vi "VSS Vision Log Player.vi"() -> ()   [LabVIEW 2018]
uses:
  GUI/IA Robot Line Display.ctl
  Intel/Functions Enum.ctl
  Filters/Estimadores.ctl
  Control/SSL Data Control.ctl
  Control/SSL UDP Address.ctl
  Control/File Player.ctl
  Intel/Command Enum.ctl
  Test/TestModule.ctl
  Util/Select None or Robot.ctl
  DrawTargets.ctl
  Select Personalitys.ctl
  Util/Select Auto None or Robot.ctl
  Intel/AI Parameters.ctl
  SSL Referee Game Status.ctl
  SSL/VSS Field State.ctl
  SSL Detection Frame.ctl
  SSL Detection Robot.ctl
  <vilib>/Analysis/Matrix/Datatypes/RealMatrix.ctl
  SSL Detection Ball.ctl
  <extravilib>/ChannelInstances/Lossy Stream-t'AI Input.ctl'/Read With Abort.vi
  <extravilib>/ChannelInstances/Lossy Stream-bool/Write With Abort.vi
  <extravilib>/ChannelInstances/Lossy Stream-a[.](u8)/Read With Abort.vi
  <extravilib>/ChannelInstances/Lossy Stream-t'VSS Field State.ctl'/Write With Abort.vi
  <extravilib>/ChannelInstances/Lossy Stream-bool/Read With Abort.vi
  <extravilib>/ChannelInstances/Lossy Stream-t'VSS Field State.ctl'/Read With Abort.vi
  <extravilib>/ChannelInstances/Lossy Stream-a[.](u16)/Write With Abort.vi
  <extravilib>/ChannelInstances/Lossy Stream-t'AI Input.ctl'/Write With Abort.vi
  <extravilib>/ChannelInstances/Lossy Stream-t'AI Input.ctl'/EndpointRead.vi
  <extravilib>/ChannelInstances/Lossy Stream-bool/Endpoint.vi
  <extravilib>/ChannelInstances/Lossy Stream-a[.](u8)/EndpointRead.vi
  <extravilib>/ChannelInstances/Lossy Stream-t'VSS Field State.ctl'/Endpoint.vi
  <extravilib>/ChannelInstances/Lossy Stream-bool/EndpointRead.vi
  <extravilib>/ChannelInstances/Lossy Stream-t'VSS Field State.ctl'/EndpointRead.vi
  <extravilib>/ChannelInstances/Lossy Stream-a[.](u16)/Endpoint.vi
  <extravilib>/ChannelInstances/Lossy Stream-t'AI Input.ctl'/Endpoint.vi
  <extravilib>/ChannelInstances/Lossy Stream-bool/Instantiate.vi
  <extravilib>/ChannelInstances/Lossy Stream-a[.](u8)/Instantiate.vi
  <extravilib>/ChannelInstances/Lossy Stream-t'VSS Field State.ctl'/Instantiate.vi
  <extravilib>/ChannelInstances/Lossy Stream-a[.](u16)/Instantiate.vi
  <extravilib>/ChannelInstances/Lossy Stream-t'AI Input.ctl'/Instantiate.vi
  <extravilib>/ChannelInstances/Lossy Stream-bool/)Channel.vi
  <resource>/ChannelSupport/_ChannelSupport/WaitIfNeeded.vi
  <extravilib>/ChannelInstances/Lossy Stream-t'VSS Field State.ctl'/)Channel.vi
  <extravilib>/ChannelInstances/Lossy Stream-a[.](u16)/)Channel.vi
  <extravilib>/ChannelInstances/Lossy Stream-t'AI Input.ctl'/)Channel.vi
  <extravilib>/ChannelInstances/Lossy Stream-a[.](u8)/)Channel.vi
  Util/PreviousState.vi
  <extravilib>/ChannelInstances/Lossy Stream-t'AI Input.ctl'.lvlib
  <extravilib>/ChannelInstances/Lossy Stream-a[.](u8).lvlib
  <vilib>/Analysis/Matrix/NI_Matrix.lvlib
  <extravilib>/ChannelInstances/Lossy Stream-t'VSS Field State.ctl'.lvlib
  <extravilib>/ChannelInstances/Lossy Stream-a[.](u16).lvlib
  <extravilib>/ChannelInstances/Lossy Stream-bool.lvlib
panel:
  in  "Personalidade Dinâmica":bool
  in  "element":T1={"Stage"="First Half", "Command"="Stop", "Time Left"=0.0, "Yellow Team"="", "Blue Team"="", "Yellow Score"=0, "Blue Score"=0, "Yellow Red Cards"=0, "Blue Red Cards"=0, "Yellow Yellow Cards"=0, "Blue Yellow Cards"=0, "Yellow Timeouts Left"=0, "Blue Timeouts Left"=0, "Yellow Timeout Remaining"=0.0, "Blue Timeout Remaining"=0.0, "Yellow Goalie Id"=0, "Blue Goalie Id"=0, "Time"=timestamp(0 s since 1904-01-01)} {"Time" format="%<%.3X %x>T"; "Blue Timeout Remaining" format="%<%M:%S>t"; "Yellow Timeout Remaining" format="%<%M:%S>t"; "Time Left" format="%<%M:%S>t"}
  in  "SSL Vision":bool
  out "Role Playing \nFPS 2":dbl
  in  "Debug":bool
  in  "GoTo Navigation":bool
  out "kick error":dbl
  in  "Pinned":T2={"Attc"="1", "Goal"="4", "Def"="2"}
  in  "Draw Targets?":T4={"Attacker"=TRUE, "Striker"=TRUE, "Goalie"=TRUE, "Defender"=TRUE, "kick"=TRUE, "Est Ball"=TRUE, "Est Robot"=FALSE, "Path S"=FALSE, "Path C"=FALSE}
  in  "SSL Data":T5={"Modo"=TRUE, "VSS Friend & ball UDP RX"={"Port:"=10006, "Server IP:"="224.5.23.2", "Local IP:"="192.168.0.101", "RX"=TRUE}, "VSS Enemy UDP RX"={"Port:"=10006, "Server IP:"="224.5.23.2", "Local IP:"="192.168.0.101", "RX"=TRUE}, "Reprodução de Arquivo"={"file path (use dialog)"=path "E:/Media/2016-07-01_cmdragons_immortals.log", "size (in bytes)"=0, "offset (in bytes)"=0, "Slide"=0.0, "Play"=FALSE, "Time Stamp"=timestamp(0 s since 1904-01-01), "Playing"=FALSE}} {"Reprodução de Arquivo"."Time Stamp" format="%<%.3X %x>T"; "Reprodução de Arquivo"."Slide" min=0 max=1 scale=0.0..1.0; "Reprodução de Arquivo"."offset (in bytes)" format="%.3p"; "Reprodução de Arquivo"."size (in bytes)" format="%.3p"}
  out "error out 5":errorcluster
  in  "IA command":T8
  in  "ignora esquerda?":bool
  in  "ignora lado?":bool
  in  "atacando ao contrário?":bool
  in  "Estimador":T9=enum."Kalman"
  out "Role Playing \nFPS":dbl
  out "Total Delay":dbl format="%#.5g"
  in  "Time":enum16{"Azul", "Amarelo"}(ring)=enum."Amarelo" caption="Enum"
  in  "Lado":enum16{"Esquerdo", "Direito"}(ring)=enum."Direito" caption="Enum"
  in  "Role Decisor":enum16{"Simple Role Decisor", "No Role Decisor"}(ring)
  out "wheel 2":dbl(graph)
  out "wheel 1":dbl(graph)
  in  "Test Module":T10={"Goto"="None", "ZigZag 0"="None", "Kicker"="None", "Vel_kick"=100.0, "Kick"=FALSE, "Modo Teste?"=FALSE, "GoTo point"=[], "zigzag points"=[{"x"=666.0, "y"=0.0}, {"x"=-666.0, "y"=0.0}], "robot id vel"=5, "Dribble"=FALSE, "Gravando"=FALSE, "output xy"=2.0, "output angle"=4.0, "angle zigzag"=0.0}
  in  "Tab Control":enum32{"RX Info", "TX info", "AI Parameters"}(tab)
  out "GUI Robot Array":T12[](array[typedef])
  in  "Serial TX":bool
  in  "UDP GrSim TX":bool=TRUE
  in  "Address:":string="192.168.0.106"
  in  "Port:":u16=10020
  in  "Porta:":refnum<visa-resource-name>
  out "Comm FPS":dbl
  in  "AI Parameters":T14={"GotoKick"={"Dist do cone a frente"=0.0, "attacker farback"=1000.0, "Perto"=300.0, "min dist to kick"=120.0, "kick eps"=0.1, "Time to transition"=0.3}, "Attacker"={"CC chute"=0.55, "CC passe"=0.4, "Kick Force"=100.0, "D ball-robot Kick"=300.0, "D ball-robot Pass"=350.0}, "Defender"={"D max"=1700.0, "Vel p/ robô av"=3.0, "Kick Force"=100.0, "D atk-def"=400.0, "D farback"=300.0}, "Timeout"={"Field/v in x"=6.0, "Dist Robots"=300, "Dist up in y"=300}, "Pose Striker"={"dist"=650.0, "Numeric"=-4.0, "dist 2"=650.0}, "Dist Stop"=300.0, "Distance when ball out"=200, "D central gap "=125.0, "T pass"=5.0, "Force ++"=100.0, "range kick"=50.0, "Chute alto"=TRUE, "Marcador novo"=TRUE} {"D central gap" format="%#_13g"; "Dist Stop" format="%#_13g"; "Pose Striker"."Numeric" format="%#_13g"; "Defender"."Kick Force" format="%#_13g"; "Defender"."Vel p/ robô av" format="%#_13g"; "Attacker"."D ball-robot Kick" format="%#_13g"; "Attacker"."Kick Force" format="%#_13g"; "Attacker"."CC passe" format="%#_13g"; "Attacker"."CC chute" format="%#_13g"; "GotoKick"."min dist to kick" format="%#_13g"; "GotoKick"."Perto" format="%#_13g"; "GotoKick"."attacker farback" format="%#_13g"; "GotoKick"."Dist do cone a frente" format="%#_13g"}
  in  "Dist posse":dbl=220.0
  in  "Tol ang posse":dbl=0.3
  in  "Dist Toque":dbl=130.0
  in  "Qtd Min p/ Stk":dbl=2.0
  # "Score"
  # "Red Cards"
  # "Yellow Cards"
  # "Timeouts Left"
  # "Timeout Remaining"
  # "Goalie ID"
  # "UDP"
  # "LOG"
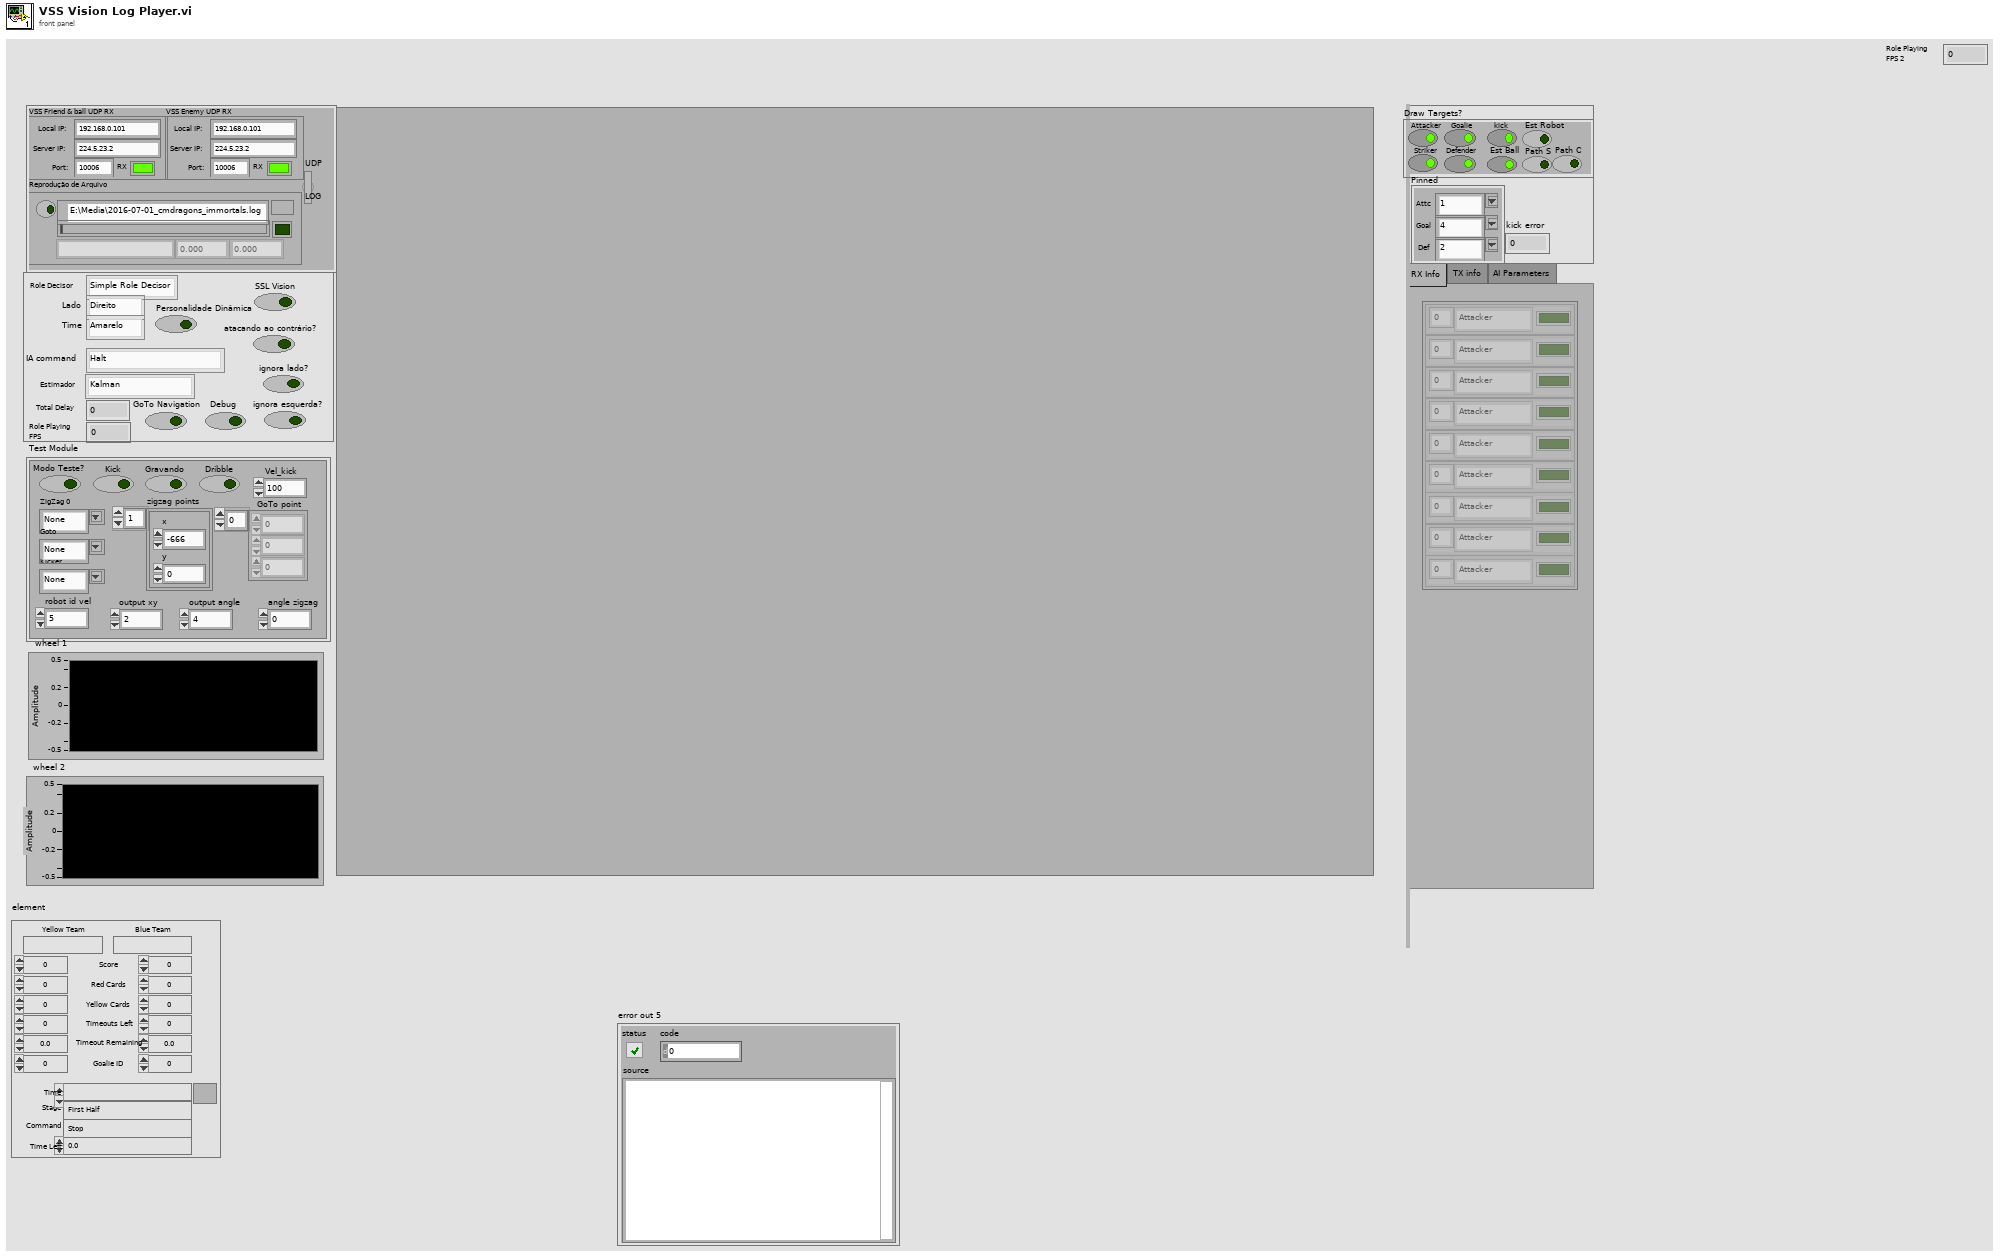
[diagram p1: front panel]
types:
  T1 = typedef "SSL Referee Game Status.ctl" = cluster{"Stage":string, "Command":string, "Time Left":dbl, "Yellow Team":string, "Blue Team":string, "Yellow Score":u32, "Blue Score":u32, "Yellow Red Cards":u32, "Blue Red Cards":u32, "Yellow Yellow Cards":u32, "Blue Yellow Cards":u32, "Yellow Timeouts Left":u32, "Blue Timeouts Left":u32, "Yellow Timeout Remaining":dbl, "Blue Timeout Remaining":dbl, "Yellow Goalie Id":u32, "Blue Goalie Id":u32, "Time":timestamp}
  T2 = typedef "Select Personalitys.ctl" = cluster{"Attc":T3, "Goal":T3, "Def":T3}
  T3 = typedef "Select Auto None or Robot.ctl" = string
  T4 = typedef "DrawTargets.ctl" = cluster{"Attacker":bool, "Striker":bool, "Goalie":bool, "Defender":bool, "kick":bool, "Est Ball":bool, "Est Robot":bool, "Path S":bool, "Path C":bool}
  T5 = typedef "SSL Data Control.ctl" = cluster{"Modo":bool, "VSS Friend & ball UDP RX":T6, "VSS Enemy UDP RX":T6, "Reprodução de Arquivo":T7}
  T6 = typedef "SSL UDP Address.ctl" = cluster{"Port:":u16, "Server IP:":string, "Local IP:":string, "RX":bool}
  T7 = typedef "File Player.ctl" = cluster{"file path (use dialog)":path, "size (in bytes)":i64, "offset (in bytes)":i64, "Slide":sgl, "Play":bool, "Time Stamp":timestamp, "Playing":bool}
  T8 = typedef "Command Enum.ctl" = enum16{"Halt", "Stop", "Force Start", "PKA Normal Start", "Prepare Kickoff Ally", "PKE Normal Start", "Prepare Kickoff Enemy", "Prepare Penalty Ally", "PPA Normal Start", "Prepare Penalty Enemy", "PPE Normal Start", "Ball Placement Enemy Up", "Ball Placement Enemy Down", "Ball Placement Ally Up", "Ball Placement Ally Mid", "Ball Placement Ally Down", "Indirect Free Enemy", "Indirect Free Ally", "Timeout Enemy", "Timeout Ally", "Goal Enemy", "Goal Ally", "Normal Half Time", "Extra Time Break", "Extra Half Time", "None", "Post Game"}
  T9 = typedef "Estimadores.ctl" = enum16{"Nenhum", "Simples", "Kalman"}
  T10 = typedef "TestModule.ctl" = cluster{"Goto":T11, "ZigZag 0":T11, "Kicker":T11, "Vel_kick":dbl, "Kick":bool, "Modo Teste?":bool, "GoTo point":dbl[], "zigzag points":cluster{"x":dbl, "y":dbl}[], "robot id vel":u32, "Dribble":bool, "Gravando":bool, "output xy":dbl, "output angle":dbl, "angle zigzag":dbl}
  T11 = typedef "Select None or Robot.ctl" = string
  T12 = typedef "IA Robot Line Display.ctl" = cluster{"ID":dbl, "function":T13, "dribble":bool}
  T13 = typedef "Functions Enum.ctl" = enum16{"Attacker", "Goalie", "Defender", "Striker", "Goto 0", "Dummy", "Kicker", "ZigZag"}
  T14 = typedef "AI Parameters.ctl" = cluster{"GotoKick":cluster{"Dist do cone a frente":dbl, "attacker farback":dbl, "Perto":dbl, "min dist to kick":dbl, "kick eps":dbl, "Time to transition":dbl}, "Attacker":cluster{"CC chute":dbl, "CC passe":dbl, "Kick Force":dbl, "D ball-robot Kick":dbl, "D ball-robot Pass":dbl}, "Defender":cluster{"D max":dbl, "Vel p/ robô av":dbl, "Kick Force":dbl, "D atk-def":dbl, "D farback":dbl}, "Timeout":cluster{"Field/v in x":dbl, "Dist Robots":u32, "Dist up in y":u32}, "Pose Striker":cluster{"dist":dbl, "Numeric":dbl, "dist 2":dbl}, "Dist Stop":dbl, "Distance when ball out":i32, "D central gap ":dbl, "T pass":dbl, "Force ++":dbl, "range kick":dbl, "Chute alto":bool, "Marcador novo":bool}
  T15 = typedef "Lossy Stream-a[.](u8).lvlib/)Channel.ctl" = refnum<queue>
  T16 = typedef "VSS Field State.ctl" = cluster{"Detection Frame Out":T17, "Received Time Stamp":timestamp, "Field Size in":cluster{"field_length":u32, "field_width":u32, "goal_width":u32, "goal_depth":u32, "center_circle_radius":u32, "defense_width":u32, "defense_depth":u32, "free_kick_from_defense_dist":u32, "penalty_spot_from_field_line_dist":u32, "penalty_line_from_spot_dist":u32, "half_moon_depth":u32, "half_moon_width":u32}}
  T17 = typedef "SSL Detection Frame.ctl" = cluster{"robots_yellow":T18[], "robots_blue":T18[], "balls":T20[], "Valid":bool, "Time Stamp":timestamp}
  T18 = typedef "SSL Detection Robot.ctl" = cluster{"x":sgl, "robot_id":u32, "confidence":sgl, "y":sgl, "orientation":sgl, "pixel_x":sgl, "pixel_y":sgl, "height":sgl, "Valid":bool, "Time Stamp":timestamp, "x_k|k":T19, "Pk|k":T19, "Previous Time Stamp":timestamp, "R":T19}
  T19 = typedef "NI_Matrix.lvlib/RealMatrix.ctl" = dbl[][]
  T20 = typedef "SSL Detection Ball.ctl" = cluster{"x":sgl, "area":u32, "confidence":sgl, "y":sgl, "z":sgl, "pixel_x":sgl, "pixel_y":sgl, "Valid":bool, "Time Stamp":timestamp, "x_k|k":T19, "Pk|k":T19, "Id":u32, "Previous Time Stamp":timestamp, "R":T19}
  T21 = typedef "VSS Geometry Field Size.ctl" = cluster{"field_length":u32, "field_width":u32, "goal_width":u32, "goal_depth":u32, "center_circle_radius":u32, "defense_width":u32, "defense_depth":u32, "free_kick_from_defense_dist":u32, "penalty_spot_from_field_line_dist":u32, "penalty_line_from_spot_dist":u32, "half_moon_depth":u32, "half_moon_width":u32}
  T22 = typedef "VSS Detection Frame.ctl" = cluster{"robots_yellow":T18[], "robots_blue":T18[], "balls":T20[], "Valid":bool, "Time Stamp":timestamp}
  T23 = typedef "Lossy Stream-bool.lvlib/)Channel.ctl" = refnum<queue>
  T24 = typedef "Lossy Stream-t'VSS Field State.ctl'.lvlib/)Channel.ctl" = refnum<queue>
  T25 = typedef "AI Input.ctl" = cluster{"our_robots":T26[], "enemy_robots":T26[], "balls":T30[], "geometry":T31, "IA Judge":T32, "Received Timestamp":timestamp, "Events":T33}
  T26 = typedef "AI Robot.ctl" = cluster{"id":u32, "function":T13, "x":dbl, "y":dbl, "orientation":dbl, "v_tangent":dbl, "v_normal":dbl, "v_ang":dbl, "kick_x":dbl, "kick_z":dbl, "dribble":bool, "Timestamp":timestamp, "estimatives":cluster{"est_v_tangent":dbl, "est_v_normal":dbl, "est_vx":dbl, "est_vy":dbl, "Pos Robot Est":dbl[]}, "dest_x_kick":dbl, "dest_y_kick":dbl, "Gap Coord":dbl[], "States":T27, "Path ":dbl[][], "Path  Smooth":dbl[][], "Dest":T28}
  T27 = typedef "AttackerStates.ctl" = enum16{"Pass", "GoToTangent", "BallGetting", "GoToKick", "Rotate anti-clockwise", "Rotate Clockwise", ""}
  T28 = typedef "PathDests.ctl" = T29[]
  T29 = typedef "PathDest.ctl" = cluster{"dest_x":dbl, "dest_y":dbl, "dest_orientation":dbl, "dest_vel":dbl}
  T30 = typedef "AI Ball.ctl" = cluster{"x":dbl, "y":dbl, "timestamp":timestamp, "Vel_x":dbl, "Vel_y":dbl, "Pos Bola Est":dbl[]}
  T31 = typedef "Field Size.ctl" = cluster{"field_length":u32, "field_width":u32, "goal_width":u32, "goal_depth":u32, "center_circle_radius":u32, "defense_width":u32, "defense_depth":u32, "free_kick_from_defense_dist":u32, "penalty_spot_from_field_line_dist":u32, "penalty_line_from_spot_dist":u32, "half_moon_depth":u32, "half_moon_width":u32}
  T32 = typedef "AI Judge.ctl" = cluster{"stage":string, "command":string, "our_goalie_id":dbl, "enemy_goalie_id":dbl, "command enum":T8, "Time":enum16{"Azul", "Amarelo"}}
  T33 = typedef "Events.ctl" = cluster{"Touch":bool, "id touch":dbl, "Ball out of \nVision":bool, "Ball inside \nGoalie area":bool, "Robot not responding":bool, "Robots responding status":dbl[], "Enemy Ball \nPossession":bool, "Id ini Possession":dbl, "Ball Possesion":bool, "Id Possesion":dbl, "Ball at\nour goal side":bool, "Ball at\ntouchline":bool, "Ball at\nenemy goal side":bool}
  T34 = typedef "Lossy Stream-a[.](u16).lvlib/)Channel.ctl" = refnum<queue>
  T35 = typedef "Lossy Stream-t'AI Input.ctl'.lvlib/)Channel.ctl" = refnum<queue>
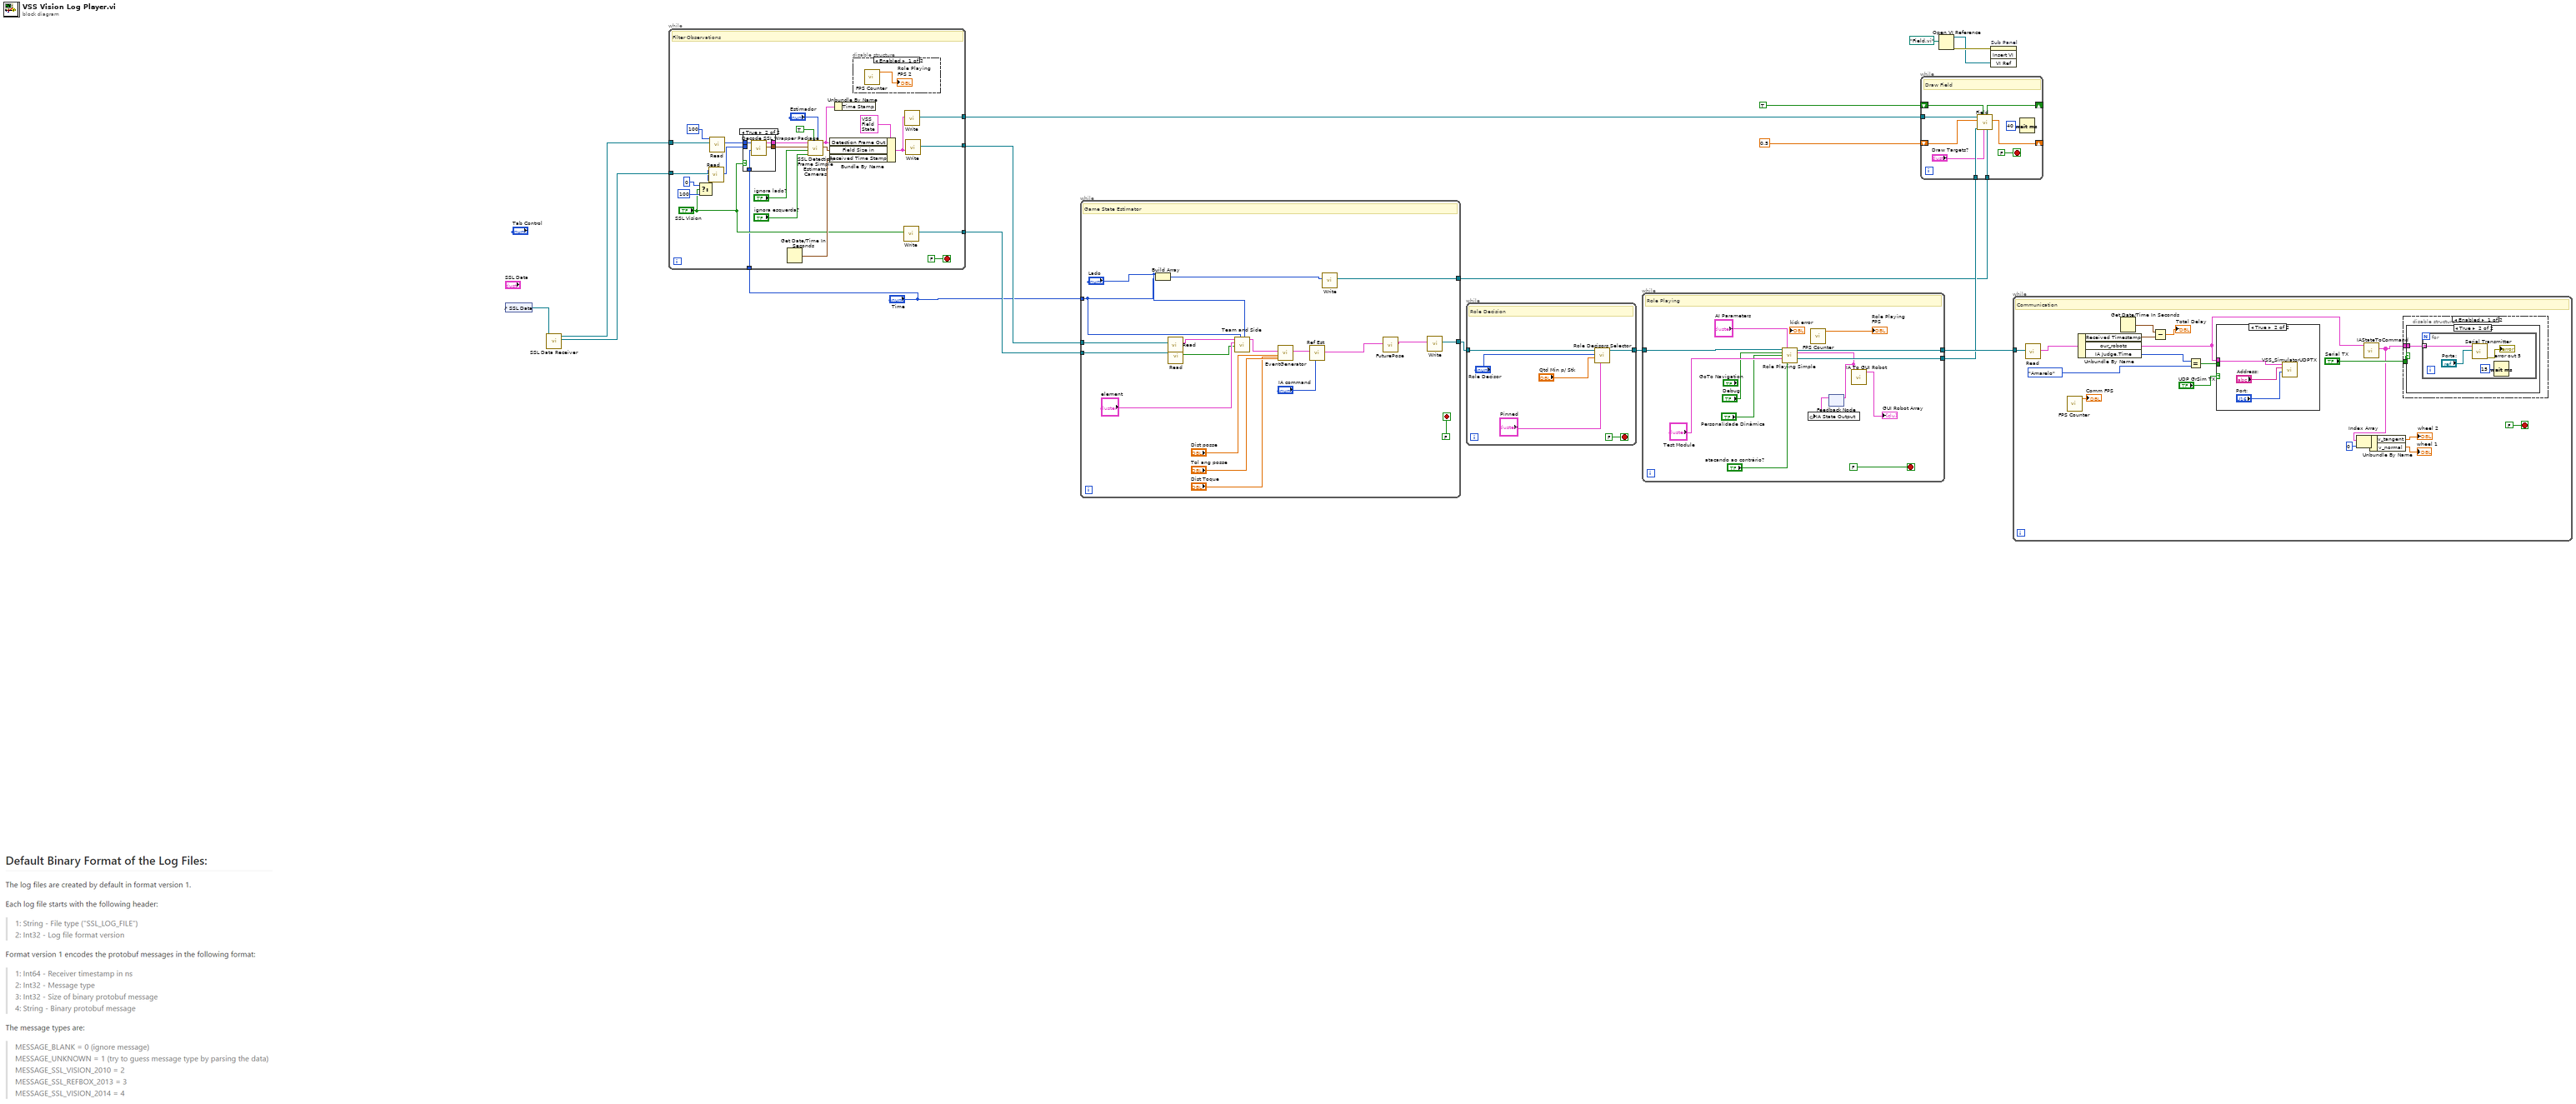
[diagram p0: block diagram]
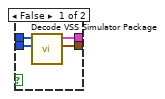
[diagram p2: hidden frame]
diagram:
  n1 = control-ref of="SSL Data"() -> (w10:refnum<vi>)
  n2 = call "SSL Data Receiver.vi"("SSL Data 2"=w10) -> ("SSL RefBox"=w3:T15, "SSL Vision"=w11:T15)  [unwired: 9 in]
  n3 = while {
    tunnel: w11 -> [w38]
    tunnel: [w31] -> w5
    tunnel: [w29] -> w4
    tunnel: w3 -> [w28]
    tunnel: [w19] -> w2
    tunnel: "Time" -> [w18]
    stop <- FALSE stop-if-true
    # "Filter Observations"
    n4 = Select(t=0 ("timeout in ms (-1)"), s="SSL Vision", f=100 ("timeout in ms (-1)")) -> (s? t:f=w21:i32)
    n5 = call <extravilib>:"Read.vi"("channel"=w28, "timeout in ms (-1)"=w21) -> ("element"=w27:u8[])  [unwired: 4 in, 5 out]
    n6 = call <extravilib>:"Read.vi"("channel"=w38, "timeout in ms (-1)"=100) -> ("element"=w37:u8[])  [unwired: 4 in, 5 out]
    n7 = case shown="True" "SSL Vision" {
      tunnel: [w46 w50] -> w41
      tunnel: w37 -> [w45 w49]
      tunnel: w27 -> [w44 _]
      tunnel: [w43 w48] -> w26
      tunnel: w18 -> [_ w47]
      frame False {
        n8 = call "Decode VSS Simulator Package.vi"("unsigned byte array 2"=w44, "unsigned byte array"=w45) -> ("Field Size out"=w43:T21, "Detection Frame"=w46:T22)  [unwired: 8 in]
      }
      frame True {
        n9 = call "Decode SSL Wrapper Package.vi"("Time"=w47, "unsigned byte array"=w49) -> ("Field Size out"=w48:T21, "Detection Frame"=w50:T17)  [unwired: 6 in, 2 out]
      }
    }
    n10 = Get Date/Time In Seconds() -> (seconds since 1Jan1904=w25:timestamp)
    n11 = call "SSL Detection Frame Simple Estimator Cameras.vi"("Estimador"="Estimador", "Enable"=TRUE, "ignora esquerda?"="ignora esquerda?", "ignora lado?"="ignora lado?", "Field Size in"=w26, "Detection Frame In"=w41) -> ("Field Size out"=w24:T21, "Detection Frame Out"=w33:T17)  [unwired: 4 in]
    n12 = Bundle By Name(cluster=T16 {"Detection Frame Out"={"robots_yellow"=[], "robots_blue"=[], "balls"=[], "Valid"=FALSE, "Time Stamp"=timestamp(0 s since 1904-01-01)}, "Received Time Stamp"=timestamp(0 s since 1904-01-01), "Field Size in"={"field_length"=1500, "field_width"=1300, "goal_width"=400, "goal_depth"=100, "center_circle_radius"=200, "defense_width"=700, "defense_depth"=150, "free_kick_from_defense_dist"=375, "penalty_spot_from_field_line_dist"=375, "penalty_line_from_spot_dist"=0, "half_moon_depth"=50, "half_moon_width"=200}}, "Detection Frame Out"=w33, "Field Size in"=w24, "Received Time Stamp"=w25) -> (w30:T16)
    n13 = Unbundle By Name(w33) -> ()  [unwired: 1 out]
    n14 = disable-structure shown="Enabled" {
      frame Enabled {
        n15 = call "FPS Counter.vi"() -> ("Numeric"=→"Role Playing \nFPS 2":dbl)  [unwired: 11 in]
      }
      frame Disabled {
      }
    }
    n16 = call <extravilib>:"Write.vi"("element"="SSL Vision") -> ("channel"=w19:T23)  [unwired: 8 in, 2 out]
    n17 = call <extravilib>:"Write.vi"("element"=w30) -> ("channel"=w29:T24)  [unwired: 8 in, 2 out]
    n18 = call <extravilib>:"Write.vi"("element"=w30) -> ("channel"=w31:T24)  [unwired: 8 in, 2 out]
  }
  n19 = while {
    tunnel: [w69] -> w9
    tunnel: [w66] -> w6
    tunnel: w5 -> [w59]
    tunnel: w2 -> [w55]
    tunnel: "Time" -> [w52]
    stop <- FALSE stop-if-true
    # "Game State Estimator"
    n20 = Build Array("Lado", w52) -> (w65:u16[])
    n21 = call <extravilib>:"Read.vi"("channel"=w59) -> ("element"=w58:T16)  [unwired: 5 in, 5 out]
    n22 = call <extravilib>:"Read.vi"("channel"=w55) -> ("element"=w54:bool)  [unwired: 5 in, 5 out]
    n23 = call "Team and Side.vi"("Lado"="Lado", "Time"=w52, "SSL Vision"=w54, "Game Status"="element", "Field State Input"=w58) -> ("IA State"=w68:T25)  [unwired: 6 in]
    n24 = call "EventGenerator.vi"("Dist Para Toque"="Dist Toque", "Tol para ang posse"="Tol ang posse", "Dist Para posse"="Dist posse", "IA State Input"=w68) -> ("IA State Output"=w67:T25)  [unwired: 7 in]
    n25 = call "Ref Est.vi"("IA command"="IA command", "IA State Input"=w67) -> ("IA State Output"=w53:T25)  [unwired: 9 in]
    n26 = call <extravilib>:"Write.vi"("element"=w65) -> ("channel"=w66:T34)  [unwired: 8 in, 2 out]
    n27 = call "FuturePose.vi"("IA State Input"=w53) -> ("output cluster"=w63:T25)  [unwired: 10 in]
    n28 = call <extravilib>:"Write.vi"("element"=w63) -> ("channel"=w69:T35)  [unwired: 8 in, 2 out]
  }
  n29 = while {
    tunnel: w9 -> [w74]
    tunnel: [w73] -> w8
    stop <- FALSE stop-if-true
    # "Role Decision"
    n30 = call "Role Decisors Selector.vi"("Pinned"="Pinned", "Qtd Min p/ Stk"="Qtd Min p/ Stk", "Role Decisor"="Role Decisor", "channel"=w74) -> ("channel"=w73:T35)  [unwired: 6 in, 1 out]
  }
  n31 = while {
    tunnel: w8 -> [w88]
    tunnel: [w87] -> w12
    tunnel: [w83] -> w7
    stop <- FALSE stop-if-true
    # "Role Playing"
    n32 = call "Role Playing Simple.vi"("channel"=w88, "AI Parameters"="AI Parameters", "Debug"="Debug", "Personalidade Dinâmica"="Personalidade Dinâmica", "test module"="Test Module", "atacando ao contrário?"="atacando ao contrário?") -> ("channel"=w87:T35, "IA State Output"=w80:T25, "channel to field"=w83:T35)  [unwired: 7 in]
    n33 = call "FPS Counter.vi"() -> ("Numeric"=→"Role Playing \nFPS":dbl)  [unwired: 11 in]
    n34 = feedback #1() -> (w81:T25)  [unwired: 1 in]
    n35 = global write "PreviousState.vi" "IA State Output"(w81) -> ()
    n36 = feedback-in #1(w80) -> ()
    n37 = call "IA To GUI Robot.vi"("Output IA"=w80) -> ("GUI Robot Array"=→"GUI Robot Array":T12[])  [unwired: 10 in]
  }
  n38 = while {
    shift-right: [w98] -> _
    shift-left: 0.5 ("New Scale") -> [w93]
    shift-right: [w97] -> _
    shift-left: TRUE ("AutoScale Out") -> [w96]
    tunnel: w7 -> [w94]
    tunnel: w6 -> [w90]
    tunnel: w4 -> [w91]
    stop <- FALSE stop-if-true
    # "Draw Field"
    n39 = call "Field.vi"("channel 2"=w90, "Draw Targets?"="Draw Targets?", "AutoScale"=w96, "channel for IA State"=w94, "Scale mm/pixel"=w93, "channel"=w91) -> ("Scale Out"=w98:dbl, "AutoScale Out"=w97:bool)  [unwired: 3 in, 1 out]
    n40 = Wait (ms)(milliseconds to wait=u32 40) -> ()  [unwired: 1 out]
  }
  n41 = Open VI Reference(vi path=path "Field.vi") -> (vi reference=w15:refnum<vi>, error out=w16:errorcluster)  [unwired: 5 in]
  n42 = invoke on="Sub Panel" class="SubPnl" method="Insert VI"(error in=w16, "VI Ref"=w15) -> ()  [unwired: 2 in, 4 out]
  n43 = while {
    tunnel: w12 -> [w116]
    stop <- FALSE stop-if-true
    # "Communication"
    n44 = call <extravilib>:"Read.vi"("channel"=w116) -> ("element"=w106:T25)  [unwired: 5 in, 5 out]
    n45 = call "FPS Counter.vi"() -> ("Numeric"=→"Comm FPS":dbl)  [unwired: 11 in]
    n46 = Unbundle By Name(w106) -> ("Received Timestamp"=w112:timestamp, "our_robots"=w105:T26[], "IA Judge.Time"=w115:enum16{"Azul", "Amarelo"})
    n47 = Get Date/Time In Seconds() -> (seconds since 1Jan1904=w111:timestamp)
    n48 = Subtract(x=w111, y=w112) -> (x-y=→"Total Delay":dbl)
    n49 = Equal?(x=w115, y=enum16{"Azul", "Amarelo"}."Amarelo") -> (x = y?=w113:bool)
    n50 = case shown="True" "UDP GrSim TX" {
      tunnel: w113 -> [_ _]
      tunnel: w105 -> [_ w125]
      frame False {
      }
      frame True {
        n51 = call "VSS_SimulatorUDPTX.vi"("Port:"="Port:", "SSL Vision Address:"="Address:", "our_robots"=w125) -> ()  [unwired: 9 in]
      }
    }
    n52 = call "IAStateToCommand.vi"("our_robots"=w105) -> ("robots out"=w104:T26[])  [unwired: 9 in, 1 out]
    n53 = Index Array(array=w104, index=0) -> (element=w103:T26)
    n54 = Unbundle By Name(w103) -> ("v_tangent"=→"wheel 2":dbl, "v_normal"=→"wheel 1":dbl)
    n55 = disable-structure shown="Enabled" {
      disable-tunnel: w104 -> [w119 _]
      disable-tunnel: "Serial TX" -> [w118 _]
      frame Enabled {
        n56 = case shown="True" w118 {
          tunnel: w119 -> [_ w120]
          frame False {
          }
          frame True {
            n57 = for {
              tunnel: w120 -> [w121] mode=indexing
              n58 = call "Serial Transmitter.vi"("Porta:"="Porta:", "Robot"=w121) -> ("error out"=→"error out 5":errorcluster)  [unwired: 9 in]
              n59 = Wait (ms)(milliseconds to wait=u32 15) -> ()  [unwired: 1 out]
            }
          }
        }
      }
      frame Disabled {
      }
    }
  }
